vi "SDSU_Registers.vi"(8 "error in (no error)":errorcluster, 9 "argument":string, 10 "action":T3(ring), 11 "file path":path=path "/home/arcconfig/DHE_RG_REGISTERS.cfg") -> (0 "error out":errorcluster, 1 "index":i32, 2 "Register":T1, 3 "Registers":T1[](array[typedef]))   [LabVIEW 2016]
uses:
  SDSU_Register.ctl
  SDSU_RegField.ctl
  <vilib>/Utility/config.llb/Read Key (String).vi
  <vilib>/Utility/config.llb/NI_LVConfig.lvlib
panel:
  in  "field":T2
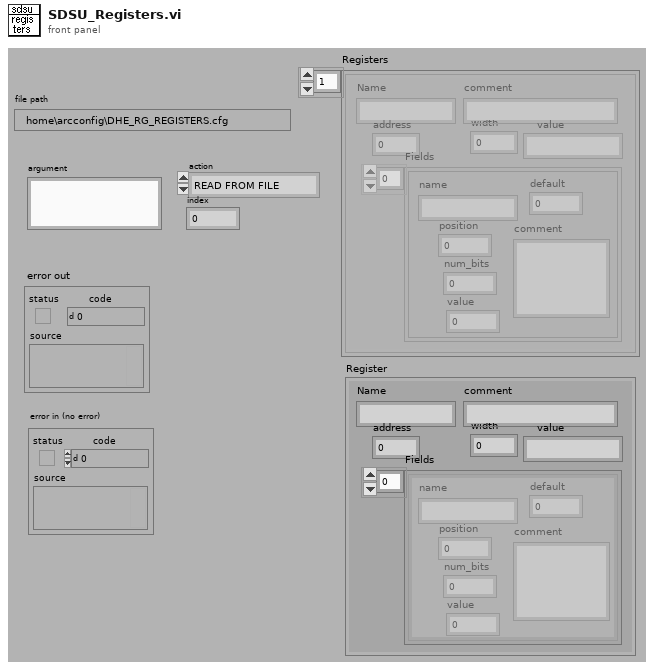
[diagram p1: front panel]
types:
  T1 = typedef "SDSU_Register.ctl" = cluster{"Name":string, "address":i16, "width":i16, "comment":string, "Fields":T2[], "value":string}
  T2 = typedef "SDSU_RegField.ctl" = cluster{"name":string, "position":u16, "num_bits":u16, "default":i16, "comment":string, "value":i32}
  T3 = enum16{"READ FROM FILE", "GET ALL", "FIND BY NAME", "SET FIELD VALUE", "CLEAN"}
  T4 = typedef "NI_LVConfig.lvlib/Config Data RefNum.ctl" = refnum<k1>
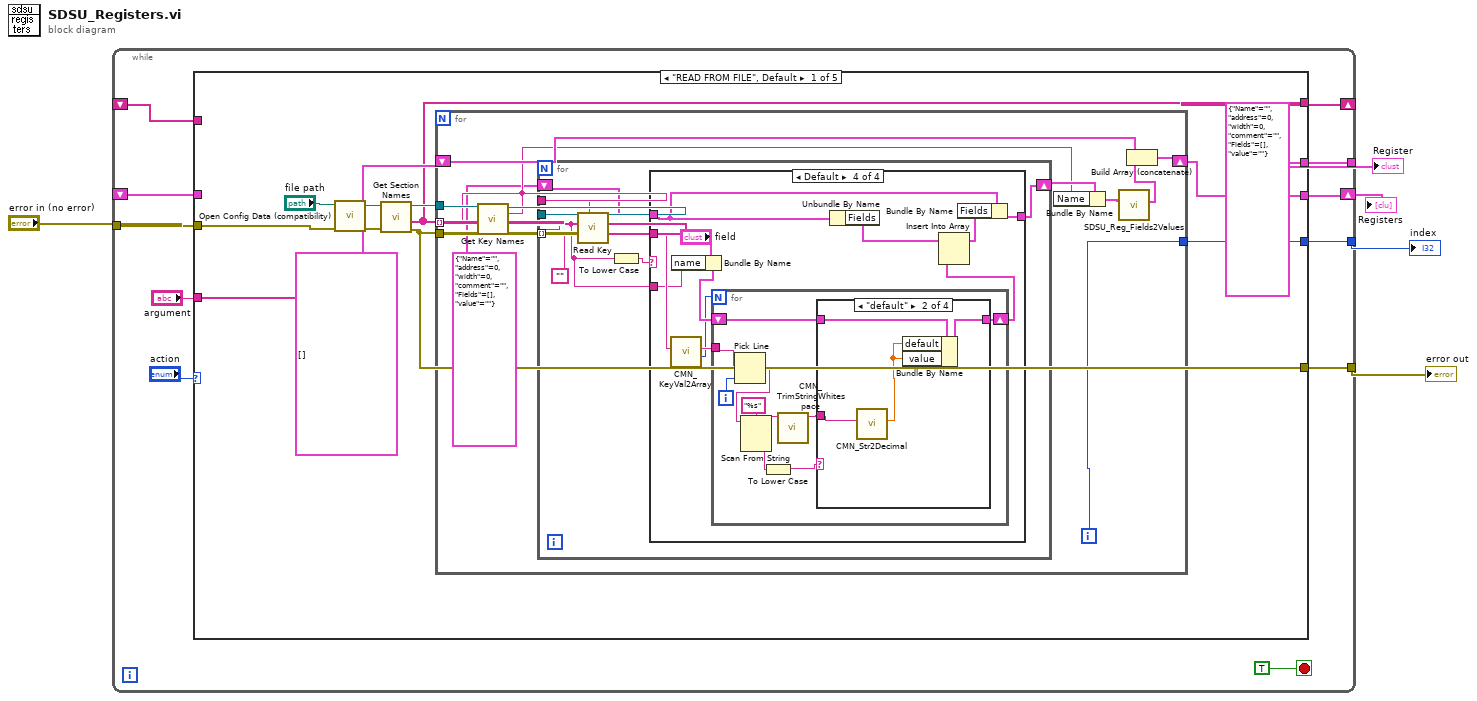
[diagram p0: block diagram]
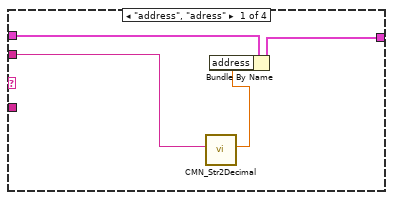
[diagram p2: hidden frame]
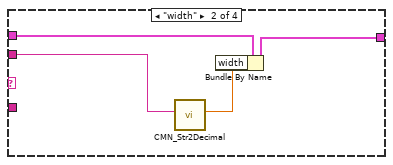
[diagram p3: hidden frame]
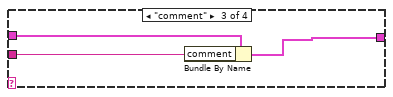
[diagram p4: hidden frame]
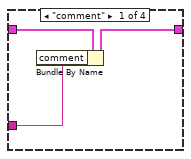
[diagram p5: hidden frame]
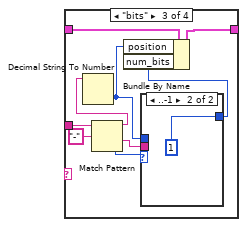
[diagram p6: hidden frame]
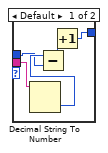
[diagram p7: hidden frame]
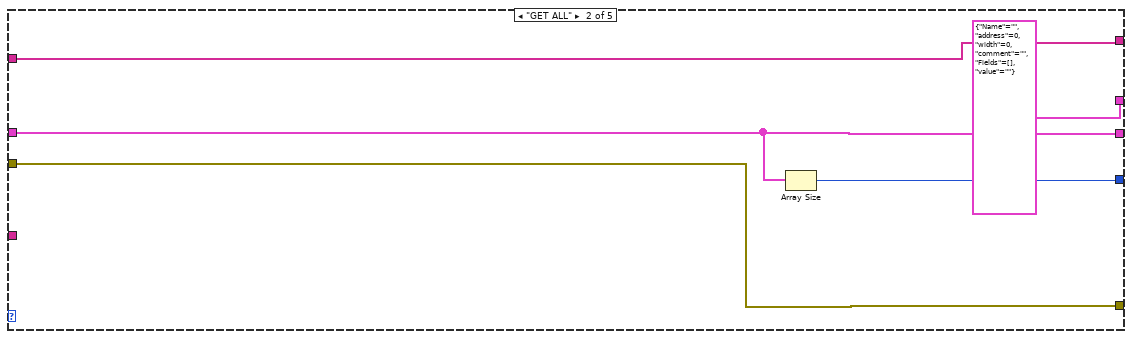
[diagram p9: hidden frame]
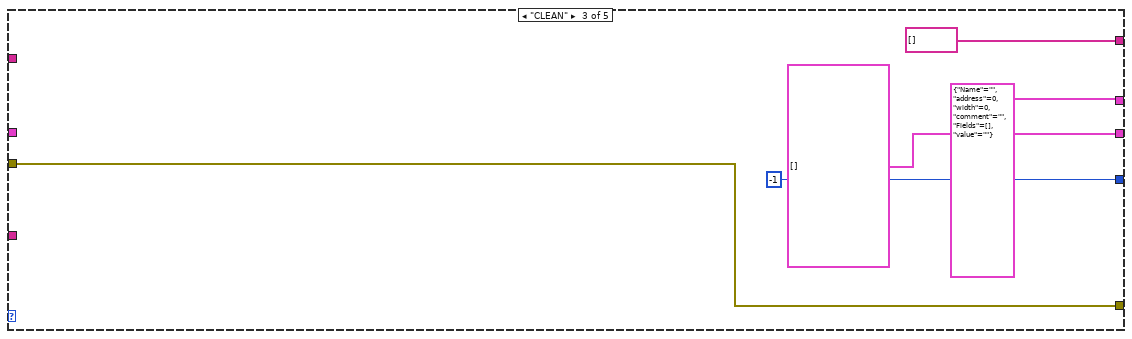
[diagram p10: hidden frame]
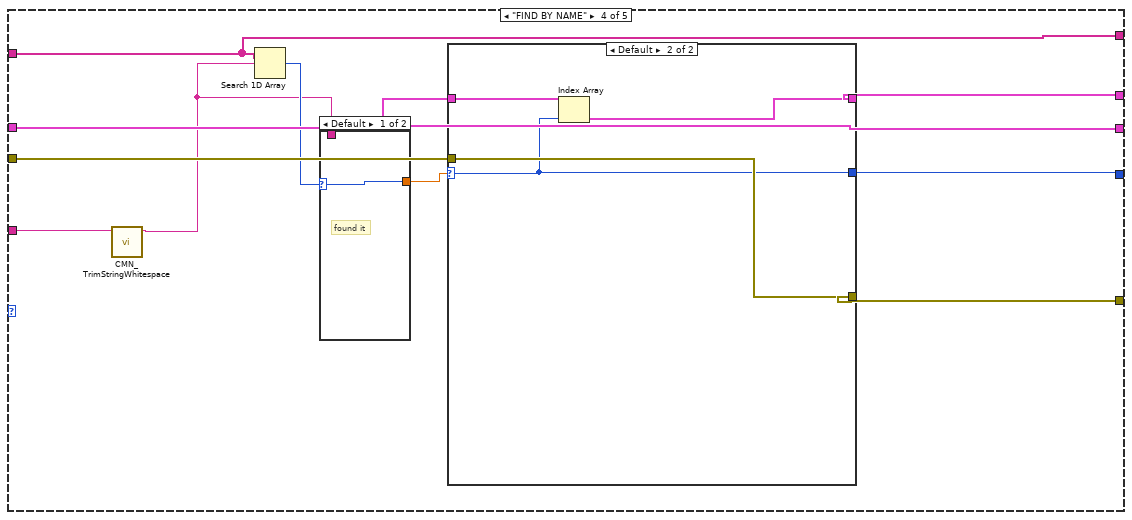
[diagram p11: hidden frame]
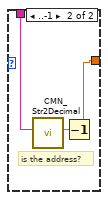
[diagram p12: hidden frame]
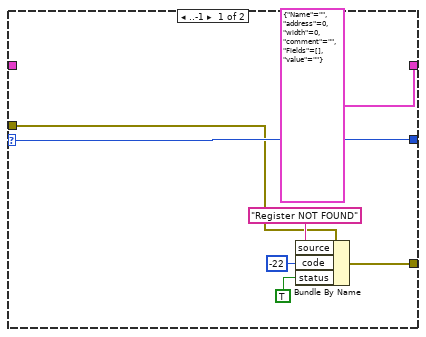
[diagram p13: hidden frame]
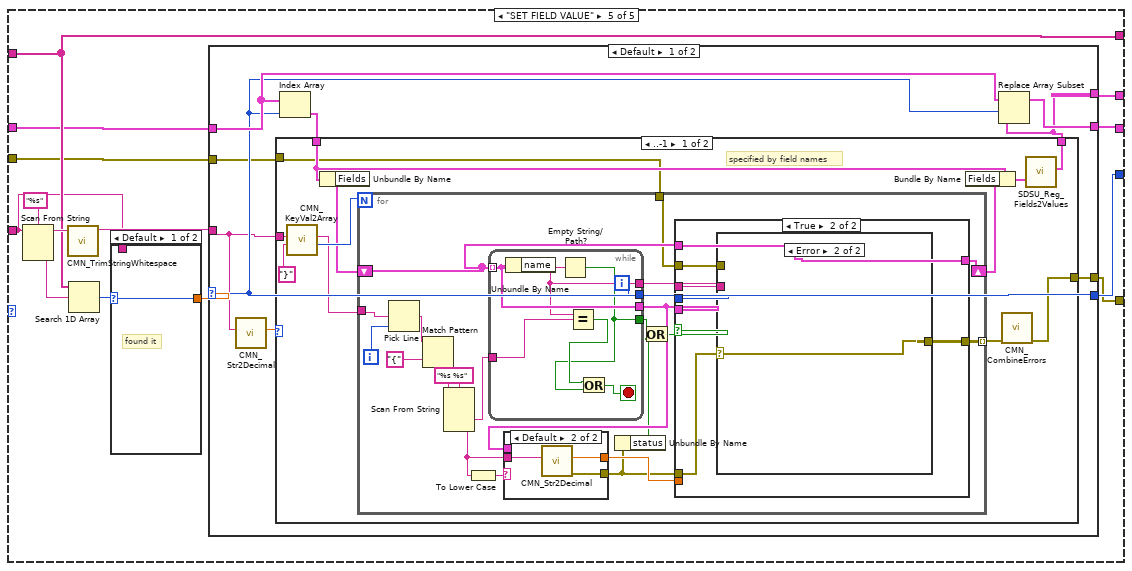
[diagram p14: hidden frame]
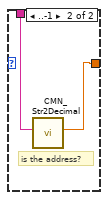
[diagram p15: hidden frame]
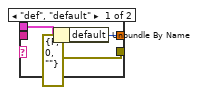
[diagram p16: hidden frame]
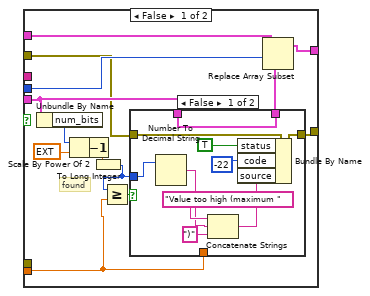
[diagram p17: hidden frame]
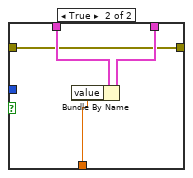
[diagram p18: hidden frame]
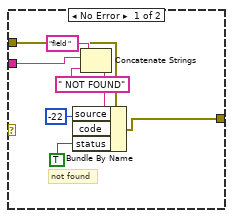
[diagram p19: hidden frame]
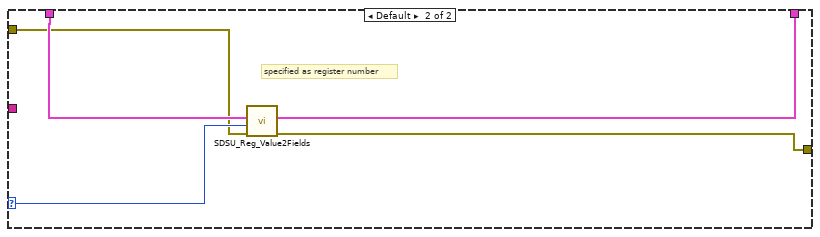
[diagram p20: hidden frame]
diagram:
  n1 = while {
    shift-right: [w13] -> w2
    shift-left: _ -> [w12]
    tunnel: "error in (no error)" -> [w14]
    tunnel: [w10] -> w4
    tunnel: [w9] -> w1
    tunnel: [w8] -> w3
    shift-right: [w7] -> _
    shift-left: _ -> [w6]
    stop <- TRUE stop-if-true
    n2 = case shown="\"READ FROM FILE\", Default" "action" {
      tunnel: w14 -> [w27 w106 w111 w121 w146]
      tunnel: [w19 w104 T1[] [] w117 w142] -> w13
      tunnel: w12 -> [_ w104 _ w117 w144]
      tunnel: "argument" -> [_ _ _ w118 w138]
      tunnel: [w23 w107 -1 ("f") w122 w147] -> w10
      tunnel: [T1 {"Name"="", "address"=0, "width"=0, "comment"="", "Fields"=[], "value"=""} ("SDSU_Register") T1 {"Name"="", "address"=0, "width"=0, "comment"="", "Fields"=[], "value"=""} ("SDSU_Register") T1 {"Name"="", "address"=0, "width"=0, "comment"="", "Fields"=[], "value"=""} ("SDSU_Register") w119 w143] -> w9
      tunnel: [w22 w106 w111 w120 w145] -> w8
      tunnel: [w20 w105 string[] [] ("section names") w116 w149] -> w7
      tunnel: w6 -> [_ w105 _ w116 w149]
      frame "READ FROM FILE", Default {
        n3 = call <vilib>:"Open Config Data (compatibility).vi"("error in (no error)"=w27, "configuration file path"="file path") -> ("error out"=w26:errorcluster, "refnum"=w25:T4)  [unwired: 7 in, 1 out]
        n4 = call <vilib>:"Get Section Names.vi"("error in (no error)"=w26, "refnum"=w25) -> ("error out"=w22:errorcluster, "section names"=w20:string[], "refnum out"=w24:T4)  [unwired: 7 out]
        n5 = for {
          tunnel: w24 -> [w39]
          tunnel: w22 -> [w38]
          tunnel: w20 -> [w31] mode=indexing
          tunnel: [w37] -> w23
          shift-right: [w36] -> w19
          shift-left: T1[] [] -> [w35]
          i -> [w37]
          n6 = call <vilib>:"Get Key Names.vi"("section"=w31, "error in (no error)"=w38, "refnum"=w39) -> ("key names"=w34:string[], "refnum out"=w33:T4)  [unwired: 7 out]
          n7 = for {
            tunnel: w34 -> [w40] mode=indexing
            tunnel: w31 -> [w46]
            tunnel: w33 -> [w45]
            shift-right: [w42] -> w32
            shift-left: T1 {"Name"="", "address"=0, "width"=0, "comment"="", "Fields"=[], "value"=""} ("SDSU_Register") -> [w41]
            n8 = call-poly <vilib>:"Read Key.vi"("section"=w46, "default value"="", "key"=w40, "refnum"=w45) -> ("value"=w43:string)  [unwired: 2 in, 5 out]
            n9 = To Lower Case(string=w40) -> (all lower case string=w47:string)
            n10 = case shown="Default" w47 {
              tunnel: w41 -> [w51 w55 w58 w68]
              tunnel: w43 -> [w49 w53 w56 w65]
              tunnel: [w50 w54 w57 w66] -> w42
              tunnel: w40 -> [_ _ _ w59]
              frame "address", "adress" {
                n11 = call "CMN_Str2Decimal.vi"("number in"=w49) -> ("decimal number"=w48:dbl)  [unwired: 1 in, 9 out]
                n12 = Bundle By Name(cluster=w51, "address"=w48) -> (w50:T1)
              }
              frame "width" {
                n13 = call "CMN_Str2Decimal.vi"("number in"=w53) -> ("decimal number"=w52:dbl)  [unwired: 1 in, 9 out]
                n14 = Bundle By Name(cluster=w55, "width"=w52) -> (w54:T1)
              }
              frame "comment" {
                n15 = Bundle By Name(cluster=w58, "comment"=w56) -> (w57:T1)
              }
              frame Default {
                n16 = call "CMN_KeyVal2Array.vi"("command in"=w65) -> ("number of commands"=w60:i32, "commands out"=w64:string)  [unwired: 2 in, 6 out]
                n17 = Bundle By Name(cluster="field", "name"=w59) -> (w62:T2)
                n18 = for {
                  N: w60 -> [_]
                  tunnel: w64 -> [w78]
                  shift-right: [w73] -> w61
                  shift-left: w62 -> [w74]
                  i -> [w79]
                  n19 = Pick Line(multi-line string=w78, line index=w79) -> (output string=w70:string)  [unwired: 1 out]
                  n20 = Scan From String(format string="%s", input string=w70) -> (remaining string=w72:string, output 1=w76:string)  [unwired: 2 in, 3 out]
                  n21 = To Lower Case(string=w76) -> (all lower case string=w75:string)
                  n22 = call "CMN_TrimStringWhitespace.vi"("string"=w72) -> ("trimmed string"=w71:string)  [unwired: 1 in, 8 out]
                  n23 = case shown="\"default\"" w75 {
                    tunnel: w74 -> [w82 w86 w92 w102]
                    tunnel: [w81 w85 w90 w102] -> w73
                    tunnel: w71 -> [w80 w84 w95 _]
                    frame "comment" {
                      n24 = Bundle By Name(cluster=w82, "comment"=w80) -> (w81:T2)
                    }
                    frame "default" {
                      n25 = call "CMN_Str2Decimal.vi"("number in"=w84) -> ("decimal number"=w83:dbl)  [unwired: 1 in, 9 out]
                      n26 = Bundle By Name(cluster=w86, "default"=w83, "value"=w83) -> (w85:T2)
                    }
                    frame "bits" {
                      n27 = Match Pattern(string=w95, regular expression="-") -> (before substring=w93:string, after substring=w89:string, offset past match=w91:i32)  [unwired: 2 out]
                      n28 = Decimal String To Number(string=w93) -> (number=w88:i32)  [unwired: 3 out]
                      n29 = case shown="..-1" w91 {
                        tunnel: w89 -> [w100 _]
                        tunnel: w88 -> [w97 _]
                        tunnel: [w96 1] -> w87
                        frame Default {
                          n30 = Decimal String To Number(string=w100) -> (number=w98:i32)  [unwired: 3 out]
                          n31 = Subtract(x=w98, y=w97) -> (x-y=w99:i32)
                          n32 = Increment(x=w99) -> (x+1=w96:i32)
                        }
                        frame ..-1 {
                        }
                      }
                      n33 = Bundle By Name(cluster=w92, "position"=w88, "num_bits"=w87) -> (w90:T2)
                    }
                    frame Default {
                    }
                  }
                }
                n34 = Unbundle By Name(w68) -> ("Fields"=w69:T2[])
                n35 = Insert Into Array(array=w69, new element=w61) -> (w67:T2[])  [unwired: 1 in]
                n36 = Bundle By Name(cluster=w68, "Fields"=w67) -> (w66:T1)
              }
            }
          }
          n37 = Bundle By Name(cluster=w32, "Name"=w31) -> (w29:T1)
          n38 = call "SDSU_Reg_Fields2Values.vi"("Register"=w29) -> ("Register out"=w28:T1)  [unwired: 10 out]
          n39 = Build Array (concatenate)(w35, w28) -> (w36:T1[])
        }
      }
      frame "GET ALL" {
        n40 = Array Size(array=w104) -> (size(s)=w107:i32)
      }
      frame "CLEAN" {
      }
      frame "FIND BY NAME" {
        n41 = call "CMN_TrimStringWhitespace.vi"("string"=w118) -> ("trimmed string"=w114:string)  [unwired: 1 in, 8 out]
        n42 = Search 1D Array(1D array=w116, element=w114) -> (index of element=w115:i32)  [unwired: 1 out]
        n43 = case shown="Default" w115 {
          selector: w115 -> [w123 _]
          tunnel: [w123 w124] -> w113
          tunnel: w114 -> [_ w126]
          frame Default {
            # "found it"
          }
          frame ..-1 {
            # "is the address?"
            n44 = call "CMN_Str2Decimal.vi"("number in"=w126) -> ("decimal number"=w125:dbl)  [unwired: 1 in, 9 out]
            n45 = Decrement(x=w125) -> (x-1=w124:dbl)
          }
        }
        n46 = case shown="Default" w113 {
          selector: w113 -> [w133 w135]
          tunnel: [w133 w135] -> w122
          tunnel: w121 -> [w130 w137]
          tunnel: [w129 w137] -> w120
          tunnel: [T1 {"Name"="", "address"=0, "width"=0, "comment"="", "Fields"=[], "value"=""} ("SDSU_Register") w134] -> w119
          tunnel: w117 -> [_ w136]
          frame ..-1 {
            n47 = Bundle By Name(cluster=w130, "source"="Register NOT FOUND", "code"=-22, "status"=TRUE) -> (w129:errorcluster)
          }
          frame Default {
            n48 = Index Array(array=w136, index=w135) -> (element=w134:T1)
          }
        }
      }
      frame "SET FIELD VALUE" {
        n49 = Scan From String(format string="%s", input string=w138) -> (remaining string=w150:string, output 1=w148:string)  [unwired: 2 in, 3 out]
        n50 = call "CMN_TrimStringWhitespace.vi"("string"=w150) -> ("trimmed string"=w139:string)  [unwired: 1 in, 8 out]
        n51 = Search 1D Array(1D array=w149, element=w148) -> (index of element=w141:i32)  [unwired: 1 out]
        n52 = case shown="Default" w141 {
          selector: w141 -> [w152 _]
          tunnel: [w152 w153] -> w140
          tunnel: w138 -> [_ w154]
          frame Default {
            # "found it"
          }
          frame ..-1 {
            # "is the address?"
            n53 = call "CMN_Str2Decimal.vi"("number in"=w154) -> ("decimal number"=w153:dbl)  [unwired: 1 in, 9 out]
          }
        }
        n54 = case shown="Default" w140 {
          selector: w140 -> [w161 _]
          tunnel: w139 -> [w156 _]
          tunnel: [w157 T1 {"Name"="", "address"=0, "width"=0, "comment"="", "Fields"=[], "value"=""} ("SDSU_Register")] -> w143
          tunnel: [w161 -1 ("f")] -> w147
          tunnel: w146 -> [w159 w262]
          tunnel: [w158 w261] -> w145
          tunnel: w144 -> [w163 w260]
          tunnel: [w162 w260] -> w142
          frame Default {
            n55 = call "CMN_Str2Decimal.vi"("number in"=w156) -> ("decimal number"=w155:dbl)  [unwired: 1 in, 9 out]
            n56 = Index Array(array=w163, index=w161) -> (element=w160:T1)
            n57 = case shown="..-1" w155 {
              selector: w155 -> [_ w255]
              tunnel: w156 -> [w175 _]
              tunnel: w160 -> [w171 w256]
              tunnel: w159 -> [w170 w253]
              tunnel: [w168 w252] -> w158
              tunnel: [w164 w254] -> w157
              frame ..-1 {
                # "specified by field names"
                n58 = call "CMN_KeyVal2Array.vi"("separator"="}", "command in"=w175) -> ("number of commands"=w174:i32, "commands out"=w166:string)  [unwired: 1 in, 6 out]
                n59 = Unbundle By Name(w171) -> ("Fields"=w173:T2[])
                n60 = for {
                  N: w174 -> [_]
                  tunnel: w166 -> [w185]
                  shift-right: [w191] -> w172
                  shift-left: w173 -> [w192]
                  tunnel: w170 -> [w190]
                  tunnel: [w188] -> w169 mode=indexing
                  i -> [w196]
                  n61 = Pick Line(multi-line string=w185, line index=w196) -> (output string=w186:string)  [unwired: 1 out]
                  n62 = Match Pattern(string=w186, regular expression="{") -> (after substring=w184:string)  [unwired: 4 out]
                  n63 = Scan From String(format string="%s %s", input string=w184) -> (output 1=w194:string, output 2=w182:string)  [unwired: 2 in, 5 out]
                  n64 = To Lower Case(string=w182) -> (all lower case string=w181:string)
                  n65 = while {
                    tunnel: w192 -> [w248] mode=indexing
                    tunnel: w194 -> [w251]
                    tunnel: [w245] -> w178
                    tunnel: [w249] -> w193
                    tunnel: [w248] -> w180
                    tunnel: [w247] -> w189
                    i -> [w249]
                    stop <- w250 stop-if-true
                    n66 = Unbundle By Name(w248) -> ("name"=w247:string)
                    n67 = Empty String/Path?(string/path=w247) -> (empty?=w245:bool)
                    n68 = Equal?(x=w247, y=w251) -> (x = y?=w246:bool)
                    n69 = Or(x=w246, y=w245) -> (x .or. y?=w250:bool)
                  }
                  n70 = case shown="Default" w181 {
                    tunnel: w182 -> [_ w202]
                    tunnel: [w198 w201] -> w183
                    tunnel: w180 -> [w199 _]
                    tunnel: [errorcluster {"status"=FALSE, "code"=0, "source"=""} ("error out") w200] -> w176
                    frame "def", "default" {
                      n71 = Unbundle By Name(w199) -> ("default"=w198:i16)
                    }
                    frame Default {
                      n72 = call "CMN_Str2Decimal.vi"("number in"=w202) -> ("error out"=w200:errorcluster, "decimal number"=w201:dbl)  [unwired: 1 in, 8 out]
                    }
                  }
                  n73 = Unbundle By Name(w176) -> ("status"=w177:bool)
                  n74 = Or(x=w178, y=w177) -> (x .or. y?=w179:bool)
                  n75 = case shown="True" w179 {
                    tunnel: w193 -> [w214 _]
                    tunnel: w192 -> [w216 w235]
                    tunnel: [w215 w235] -> w191
                    tunnel: w180 -> [w213 _]
                    tunnel: w183 -> [w209 _]
                    tunnel: w190 -> [w206 w232]
                    tunnel: w189 -> [_ w234]
                    tunnel: [w205 w233] -> w188
                    tunnel: w176 -> [_ w231]
                    frame False {
                      # "found"
                      n76 = Unbundle By Name(w213) -> ("num_bits"=w212:u16)
                      n77 = Scale By Power Of 2(n=w212, x=ext 1.0) -> (x*2^n=w210:ext)
                      n78 = Decrement(x=w210) -> (x-1=w203:ext)
                      n79 = To Long Integer(number=w203) -> (32bit integer=w204:i32)
                      n80 = Greater Or Equal?(x=w204, y=w209) -> (x >= y?=w208:bool)
                      n81 = case shown="False" w208 {
                        tunnel: w213 -> [w217 w230]
                        tunnel: w209 -> [_ w229]
                        tunnel: [w217 w228] -> w207
                        tunnel: [w225 w227] -> w205
                        tunnel: w206 -> [w226 w227]
                        tunnel: w204 -> [w222 _]
                        frame False {
                          n82 = Number To Decimal String(number=w222) -> (decimal integer string=w220:string)  [unwired: 1 out]
                          n83 = Concatenate Strings("Value too high (maximum " ("source"), w220, ")" ("string")) -> (w218:string)
                          n84 = Bundle By Name(cluster=w226, "status"=TRUE, "code"=-22, "source"=w218) -> (w225:errorcluster)
                        }
                        frame True {
                          n85 = Bundle By Name(cluster=w230, "value"=w229) -> (w228:T2)
                        }
                      }
                      n86 = Replace Array Subset(array=w216, new element=w207, index=w214) -> (w215:T2[])
                    }
                    frame True {
                      n87 = case shown="Error" w231 {
                        selector: w231 -> [_ w244]
                        tunnel: w234 -> [w239 _]
                        tunnel: [w238 w244] -> w233
                        tunnel: w232 -> [w237 _]
                        frame No Error {
                          # "not found"
                          n88 = Concatenate Strings("field ", w239, " NOT FOUND" ("source")) -> (w241:string)
                          n89 = Bundle By Name(cluster=w237, "source"=w241, "code"=-22, "status"=TRUE) -> (w238:errorcluster)
                        }
                        frame Error {
                        }
                      }
                    }
                  }
                }
                n90 = Bundle By Name(cluster=w171, "Fields"=w172) -> (w165:T1)
                n91 = call "CMN_CombineErrors.vi"("Errors"=w169) -> ("error out"=w168:errorcluster)  [unwired: 10 out]
                n92 = call "SDSU_Reg_Fields2Values.vi"("Register"=w165) -> ("Register out"=w164:T1)  [unwired: 10 out]
              }
              frame Default {
                # "specified as register number"
                n93 = call "SDSU_Reg_Value2Fields.vi"("error in (no error)"=w253, "value"=w255, "Register"=w256) -> ("error out"=w252:errorcluster, "Register out"=w254:T1)  [unwired: 7 out]
              }
            }
            n94 = Replace Array Subset(array=w163, new element=w157, index=w161) -> (w162:T1[])
          }
          frame ..-1 {
            n95 = Bundle By Name(cluster=w262, "source"="Register NOT FOUND", "code"=-22, "status"=TRUE) -> (w261:errorcluster)
          }
        }
      }
    }
  }
  "error out" <- w3
  "index" <- w4
  "Registers" <- w2
  "Register" <- w1
